vi "cost_so_far.vi"(10 "Node":cluster{"Weight":dbl, "Row":dbl, "Col":dbl}, 11 "Cost_so_far":T1(array[cluster])) -> (3 "cost out":dbl)   [LabVIEW 2014]
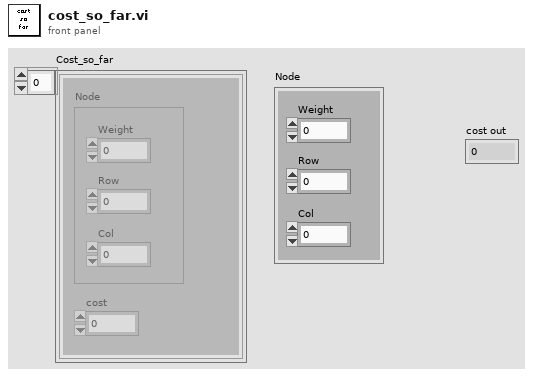
[diagram p1: front panel]
types:
  T1 = cluster{"Node":cluster{"Weight":dbl, "Row":dbl, "Col":dbl}, "cost":dbl}[]
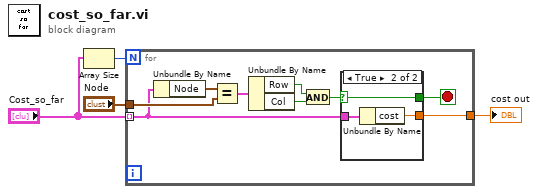
[diagram p0: block diagram]
diagram:
  n1 = Array Size(array="Cost_so_far") -> (size(s)=w4:i32)
  n2 = for {
    N: w4 -> [_]
    tunnel: "Node" -> [w12]
    tunnel: "Cost_so_far" -> [w11] mode=indexing
    tunnel: [w10] -> w1
    stop <- w9 stop-if-true
    n3 = Unbundle By Name(w11) -> ("Node"=w13:cluster{"Weight":dbl, "Row":dbl, "Col":dbl})
    n4 = Equal?(x=w13, y=w12) -> (x = y?=w8:cluster{"Weight":bool, "Row":bool, "Col":bool})
    n5 = Unbundle By Name(w8) -> ("Row"=w7:bool, "Col"=w6:bool)
    n6 = And(x=w7, y=w6) -> (x .and. y?=w5:bool)
    n7 = case shown="True" w5 {
      selector: w5 -> [w14 w15]
      tunnel: w11 -> [_ w17]
      tunnel: [_ w16] -> w10
      tunnel: [w14 w15] -> w9
      frame False {
      }
      frame True {
        n8 = Unbundle By Name(w17) -> ("cost"=w16:dbl)
      }
    }
  }
  "cost out" <- w1
